vi "Write Attributes.vi"(4 "Attributes":variant[](array[variant]), 6 "Attribute Names":string[](array[string]), 11 "Executioner in":refnum<class "Executioner.lvclass">) -> (3 "Executioner out":refnum<class "Executioner.lvclass">)   [LabVIEW 2017, in "Test Executive.lvlib" / "Executioner.lvclass"]
uses:
  <vilib>/gpm_packages/@cs/test-executive/Source/Test Executive/Executioner/Executioner.lvclass
  <vilib>/gpm_packages/@cs/test-executive/Source/Test Executive/Executioner/Executioner.lvclass/Executioner.ctl
  <vilib>/gpm_packages/@cs/lookup-table/Source/LookupTable/LookupTable.lvclass/LookupTable.ctl
  72db7eac-e962-4688-b52f-1e20fe5ff9a1.vi
  <vilib>/gpm_packages/@cs/lookup-table/Source/LookupTable/Read Table Reference.vi
  72db7eac-e962-4688-b52f-1e20fe5ff9a1.vi/08af0801-b87b-44ba-8ce4-f0b7c7c5af96.vi
  <vilib>/gpm_packages/@cs/lookup-table/Source/LookupTable/LookupTable.lvclass
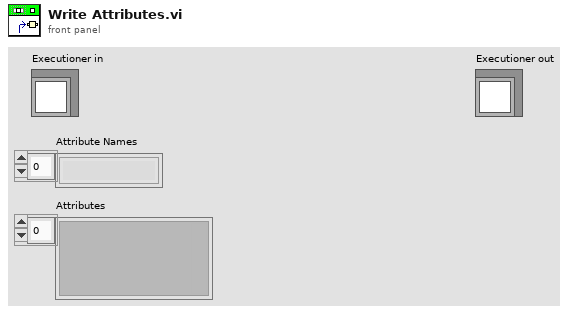
[diagram p1: front panel]
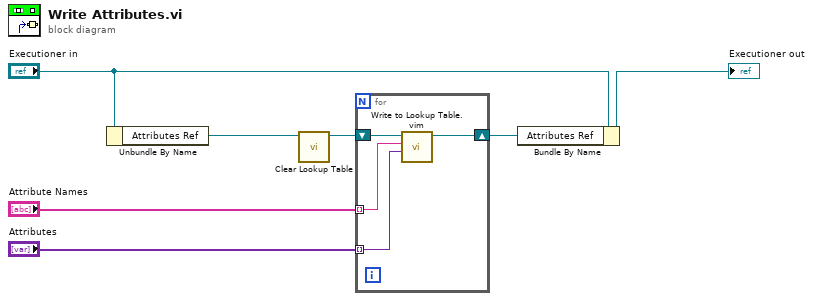
[diagram p0: block diagram]
diagram:
  n1 = Unbundle By Name("Executioner in") -> ("Attributes Ref"=w7:refnum<data-value>)
  n2 = call <vilib>:"Clear Lookup Table.vi"("LookupTable Reference"=w7) -> ("LookupTable Reference Out"=w6:refnum<data-value>)  [unwired: 9 in, 1 out]
  n3 = for {
    shift-right: [w10] -> w3
    shift-left: w6 -> [w11]
    tunnel: "Attribute Names" -> [w9] mode=indexing
    tunnel: "Attributes" -> [w8] mode=indexing
    n4 = call "Write to Lookup Table.vim"("Item"=w8, "Item Name"=w9, "LookupTable Reference"=w11) -> ("LookupTable Reference Out"=w10:refnum<data-value>)  [unwired: 6 in, 2 out]
  }
  n5 = Bundle By Name(cluster="Executioner in", "Attributes Ref"=w3) -> (→"Executioner out":refnum<class "Executioner.lvclass">)
